vi "Read Event Log Credentials.vi"(11 "IMediator in":refnum<class "IMediator.lvclass">) -> (1 "Framework Instance Alias":string, 2 "Event Log Instance":refnum<class "LoggerReference.lvclass">)   [LabVIEW 2020, in "IMediator.lvlib" / "IMediator.lvclass"]
uses:
  <vilib>/gpm_packages/@cs/mva-core/Source/IMediator/IMediator/IMediator.lvclass
  <vilib>/gpm_packages/@cs/event-logger/Source/Composed Log/LoggerReference/LoggerReference.lvclass
  <vilib>/gpm_packages/@cs/mva-core/Source/IMediator/IMediator/IMediator.lvclass/IMediator.ctl
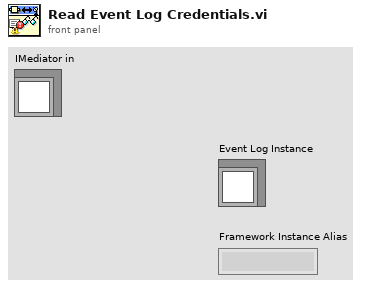
[diagram p1: front panel]
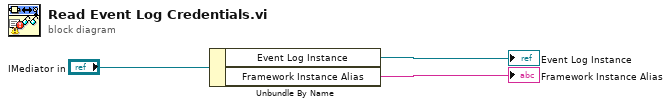
[diagram p0: block diagram]
diagram:
  n1 = Unbundle By Name("IMediator in") -> ("Event Log Instance"=→"Event Log Instance":refnum<class "LoggerReference.lvclass">, "Framework Instance Alias"=→"Framework Instance Alias":string)
